vi "CAN_Frame.vi"() -> (3 "appended array":T1(array[cluster]))   [LabVIEW 2026]
panel:
  in  "CAN FRAME":T2
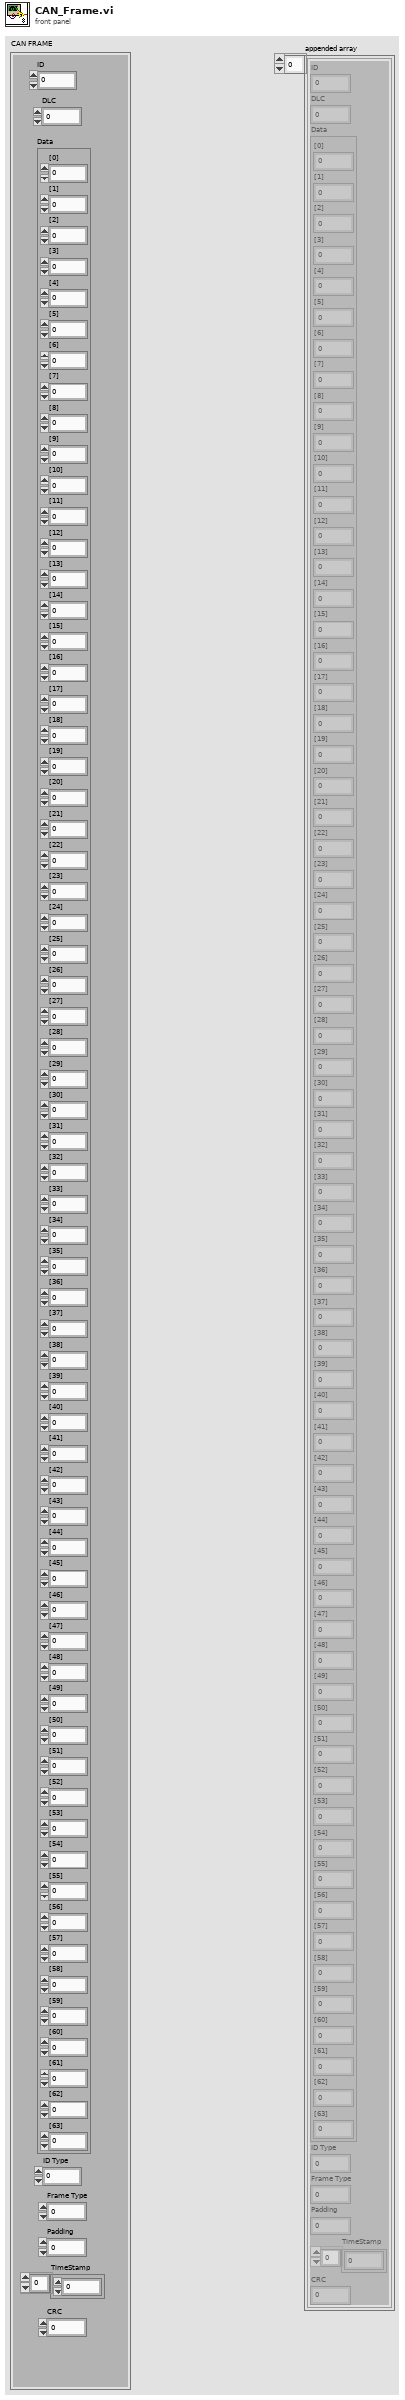
[diagram p1: front panel]
types:
  T1 = cluster{"ID":u32, "DLC":u8, "Data":cluster{"[0]":u8, "[1]":u8, "[2]":u8, "[3]":u8, "[4]":u8, "[5]":u8, "[6]":u8, "[7]":u8, "[8]":u8, "[9]":u8, "[10]":u8, "[11]":u8, "[12]":u8, "[13]":u8, "[14]":u8, "[15]":u8, "[16]":u8, "[17]":u8, "[18]":u8, "[19]":u8, "[20]":u8, "[21]":u8, "[22]":u8, "[23]":u8, "[24]":u8, "[25]":u8, "[26]":u8, "[27]":u8, "[28]":u8, "[29]":u8, "[30]":u8, "[31]":u8, "[32]":u8, "[33]":u8, "[34]":u8, "[35]":u8, "[36]":u8, "[37]":u8, "[38]":u8, "[39]":u8, "[40]":u8, "[41]":u8, "[42]":u8, "[43]":u8, "[44]":u8, "[45]":u8, "[46]":u8, "[47]":u8, "[48]":u8, "[49]":u8, "[50]":u8, "[51]":u8, "[52]":u8, "[53]":u8, "[54]":u8, "[55]":u8, "[56]":u8, "[57]":u8, "[58]":u8, "[59]":u8, "[60]":u8, "[61]":u8, "[62]":u8, "[63]":u8}, "ID Type":u8, "Frame Type":u8, "Padding":u8, "TimeStamp":u8[], "CRC":u16}[]
  T2 = cluster{"ID":u32, "DLC":u8, "Data":cluster{"[0]":u8, "[1]":u8, "[2]":u8, "[3]":u8, "[4]":u8, "[5]":u8, "[6]":u8, "[7]":u8, "[8]":u8, "[9]":u8, "[10]":u8, "[11]":u8, "[12]":u8, "[13]":u8, "[14]":u8, "[15]":u8, "[16]":u8, "[17]":u8, "[18]":u8, "[19]":u8, "[20]":u8, "[21]":u8, "[22]":u8, "[23]":u8, "[24]":u8, "[25]":u8, "[26]":u8, "[27]":u8, "[28]":u8, "[29]":u8, "[30]":u8, "[31]":u8, "[32]":u8, "[33]":u8, "[34]":u8, "[35]":u8, "[36]":u8, "[37]":u8, "[38]":u8, "[39]":u8, "[40]":u8, "[41]":u8, "[42]":u8, "[43]":u8, "[44]":u8, "[45]":u8, "[46]":u8, "[47]":u8, "[48]":u8, "[49]":u8, "[50]":u8, "[51]":u8, "[52]":u8, "[53]":u8, "[54]":u8, "[55]":u8, "[56]":u8, "[57]":u8, "[58]":u8, "[59]":u8, "[60]":u8, "[61]":u8, "[62]":u8, "[63]":u8}, "ID Type":u8, "Frame Type":u8, "Padding":u8, "TimeStamp":u8[], "CRC":u16}
  T3 = cluster{"initialized array[0]":u8, "initialized array[1]":u8, "initialized array[2]":u8, "initialized array[3]":u8, "initialized array[4]":u8, "initialized array[5]":u8, "initialized array[6]":u8, "initialized array[7]":u8, "initialized array[8]":u8, "initialized array[9]":u8, "initialized array[10]":u8, "initialized array[11]":u8, "initialized array[12]":u8, "initialized array[13]":u8, "initialized array[14]":u8, "initialized array[15]":u8, "initialized array[16]":u8, "initialized array[17]":u8, "initialized array[18]":u8, "initialized array[19]":u8, "initialized array[20]":u8, "initialized array[21]":u8, "initialized array[22]":u8, "initialized array[23]":u8, "initialized array[24]":u8, "initialized array[25]":u8, "initialized array[26]":u8, "initialized array[27]":u8, "initialized array[28]":u8, "initialized array[29]":u8, "initialized array[30]":u8, "initialized array[31]":u8, "initialized array[32]":u8, "initialized array[33]":u8, "initialized array[34]":u8, "initialized array[35]":u8, "initialized array[36]":u8, "initialized array[37]":u8, "initialized array[38]":u8, "initialized array[39]":u8, "initialized array[40]":u8, "initialized array[41]":u8, "initialized array[42]":u8, "initialized array[43]":u8, "initialized array[44]":u8, "initialized array[45]":u8, "initialized array[46]":u8, "initialized array[47]":u8, "initialized array[48]":u8, "initialized array[49]":u8, "initialized array[50]":u8, "initialized array[51]":u8, "initialized array[52]":u8, "initialized array[53]":u8, "initialized array[54]":u8, "initialized array[55]":u8, "initialized array[56]":u8, "initialized array[57]":u8, "initialized array[58]":u8, "initialized array[59]":u8, "initialized array[60]":u8, "initialized array[61]":u8, "initialized array[62]":u8, "initialized array[63]":u8}
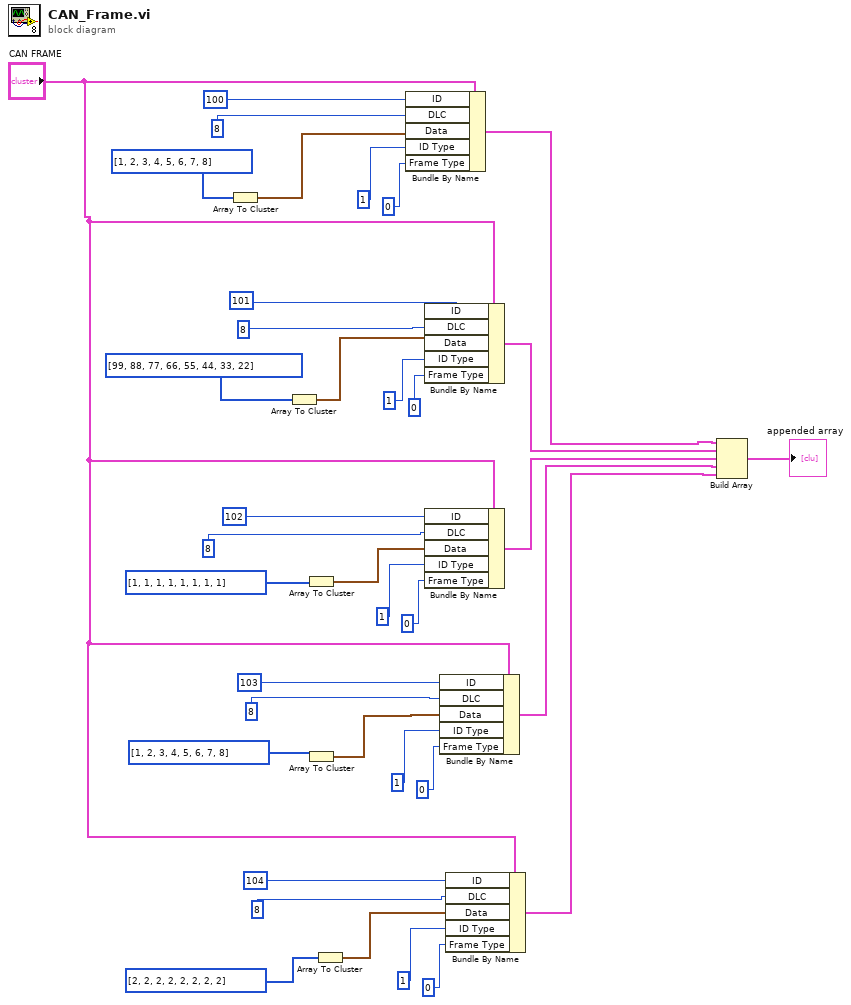
[diagram p0: block diagram]
diagram:
  n1 = Array To Cluster(array=u8[] [1, 2, 3, 4, 5, 6, 7, 8] ("initialized array")) -> (cluster=w25:T3)
  n2 = Array To Cluster(array=u8[] [99, 88, 77, 66, 55, 44, 33, 22] ("initialized array")) -> (cluster=w20:T3)
  n3 = Array To Cluster(array=u8[] [1, 1, 1, 1, 1, 1, 1, 1] ("initialized array")) -> (cluster=w6:T3)
  n4 = Array To Cluster(array=u8[] [1, 2, 3, 4, 5, 6, 7, 8] ("initialized array")) -> (cluster=w8:T3)
  n5 = Array To Cluster(array=u8[] [2, 2, 2, 2, 2, 2, 2, 2] ("initialized array")) -> (cluster=w10:T3)
  n6 = Bundle By Name(cluster="CAN FRAME", "ID"=100, "DLC"=8, "Data"=w25, "ID Type"=1, "Frame Type"=0) -> (w5:T2)
  n7 = Bundle By Name(cluster="CAN FRAME", "ID"=101, "DLC"=8, "Data"=w20, "ID Type"=1, "Frame Type"=0) -> (w19:T2)
  n8 = Bundle By Name(cluster="CAN FRAME", "ID"=102, "DLC"=8, "Data"=w6, "ID Type"=1, "Frame Type"=0) -> (w4:T2)
  n9 = Bundle By Name(cluster="CAN FRAME", "ID"=103, "DLC"=8, "Data"=w8, "ID Type"=1, "Frame Type"=0) -> (w3:T2)
  n10 = Bundle By Name(cluster="CAN FRAME", "ID"=104, "DLC"=8, "Data"=w10, "ID Type"=1, "Frame Type"=0) -> (w2:T2)
  n11 = Build Array(w5, w19, w4, w3, w2) -> (→"appended array":T1)
